vi "Load Sensors.vi"(8 "error in (no error)":errorcluster, 10 "refnum":T1, 11 "Sensor List Class in":refnum<class "Sensor List Class.lvclass">) -> (0 "error out":errorcluster, 2 "refnum out":T1, 3 "Sensor List Class out":refnum<class "Sensor List Class.lvclass">)   [LabVIEW 2013, in "Sensor List Class.lvclass"]
uses:
  Sensor List Class.lvclass
  <vilib>/Utility/config.llb/Config Data RefNum.ctl
  Sensor DAO Class.lvclass
  Sensor List Class.lvclass/Sensor List Class.ctl
  Sensor DAO Class.lvclass/Sensor DAO Class.ctl
  <vilib>/Utility/config.llb/NI_LVConfig.lvlib
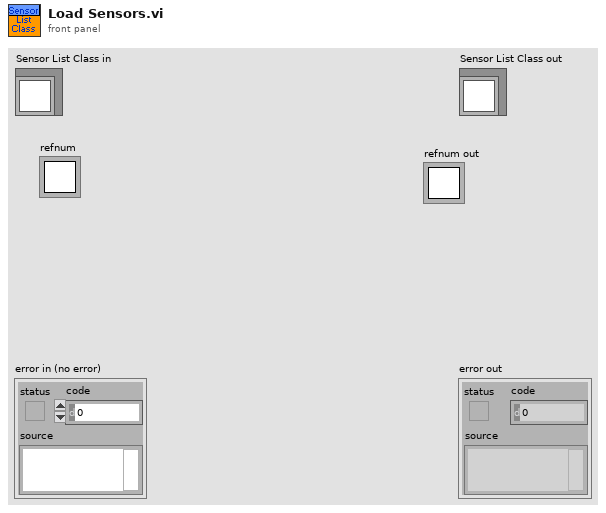
[diagram p1: front panel]
types:
  T1 = typedef "NI_LVConfig.lvlib/Config Data RefNum.ctl" = refnum<k1>
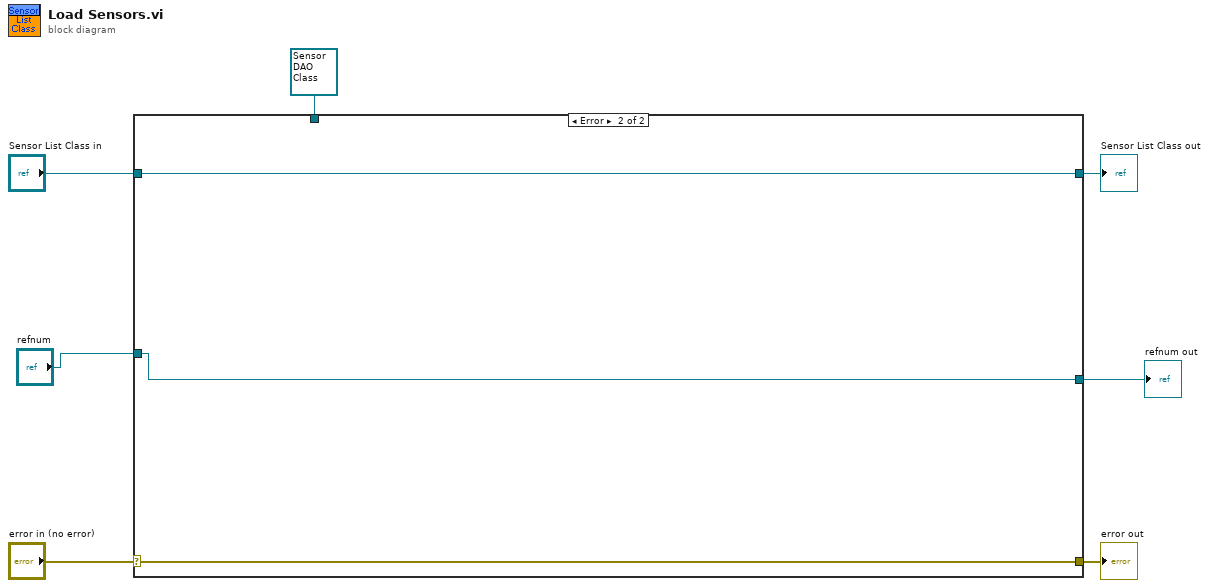
[diagram p0: block diagram]
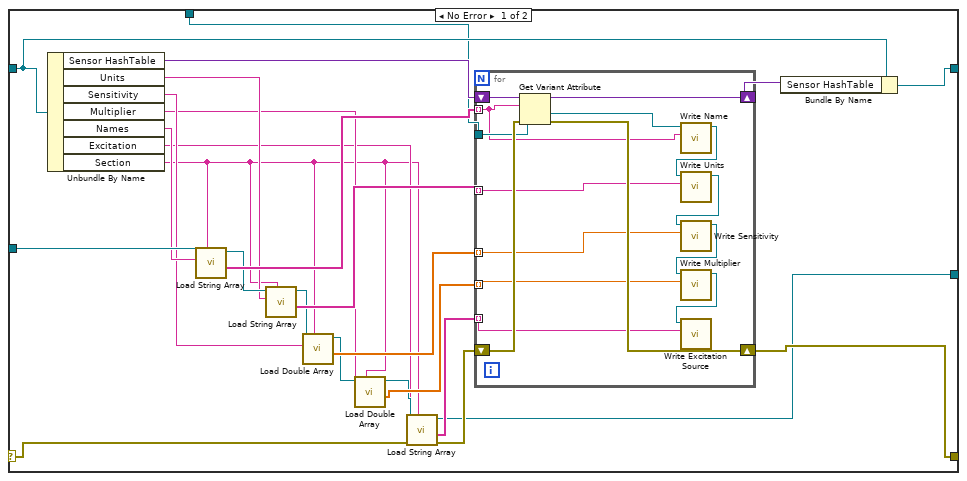
[diagram p2: hidden frame]
diagram:
  n1 = case shown="Error" "error in (no error)" {
    selector: "error in (no error)" -> [w22 w50]
    tunnel: [w21 w50] -> w6
    tunnel: [w18 w49] -> w4
    tunnel: "Sensor List Class in" -> [w20 w49]
    tunnel: "refnum" -> [w15 w48]
    tunnel: [w14 w48] -> w2
    tunnel: refnum<class "Sensor DAO Class.lvclass"> refnum ("Sensor DAO In") -> [w9 _]
    frame No Error {
      n2 = Unbundle By Name(w20) -> ("Sensor HashTable"=w19:variant, "Units"=w16:string, "Sensitivity"=w12:string, "Multiplier"=w11:string, "Names"=w13:string, "Excitation"=w10:string, "Section"=w8:string)
      n3 = call "Load String Array.vi"("section"=w8, "key"=w13, "refnum"=w15) -> ("String Array Out"=w27:string[], "refnum out"=w23:T1)  [unwired: 6 in, 1 out]
      n4 = call "Load String Array.vi"("section"=w8, "key"=w16, "refnum"=w23) -> ("String Array Out"=w28:string[], "refnum out"=w24:T1)  [unwired: 6 in, 1 out]
      n5 = call "Load Double Array.vi"("section"=w8, "key"=w12, "refnum"=w24) -> ("String Array Out"=w29:dbl[], "refnum out"=w25:T1)  [unwired: 6 in, 1 out]
      n6 = call "Load Double Array.vi"("section"=w8, "key"=w11, "refnum"=w25) -> ("String Array Out"=w30:dbl[], "refnum out"=w26:T1)  [unwired: 6 in, 1 out]
      n7 = call "Load String Array.vi"("section"=w8, "error in (no error)"=w22, "key"=w10, "refnum"=w26) -> ("error out"=w32:errorcluster, "String Array Out"=w31:string[], "refnum out"=w14:T1)  [unwired: 5 in]
      n8 = for {
        shift-right: [w46] -> w17
        shift-left: w19 -> [w47]
        shift-right: [w43] -> w21
        shift-left: w32 -> [w44]
        tunnel: w27 -> [w40] mode=indexing
        tunnel: w9 -> [w42]
        tunnel: w28 -> [w41] mode=indexing
        tunnel: w29 -> [w39] mode=indexing
        tunnel: w30 -> [w38] mode=indexing
        tunnel: w31 -> [w37] mode=indexing
        n9 = Get Variant Attribute(Variant=w47, name=w40, default value (empty Variant)=w42, error in=w44) -> (duplicate Variant=w46:variant, value=w45:refnum<class "Sensor DAO Class.lvclass">, error out=w43:errorcluster)  [unwired: 1 out]
        n10 = call "Write Name.vi"("Name"=w40, "Sensor DAO Class in"=w45) -> ("Sensor DAO Class out"=w36:refnum<class "Sensor DAO Class.lvclass">)  [unwired: 8 in, 1 out]
        n11 = call "Write Units.vi"("Units"=w41, "Sensor DAO Class in"=w36) -> ("Sensor DAO Class out"=w35:refnum<class "Sensor DAO Class.lvclass">)  [unwired: 8 in, 1 out]
        n12 = call "Write Sensitivity.vi"("Sensitivity"=w39, "Sensor DAO Class in"=w35) -> ("Sensor DAO Class out"=w34:refnum<class "Sensor DAO Class.lvclass">)  [unwired: 8 in, 1 out]
        n13 = call "Write Multiplier.vi"("Multiplier"=w38, "Sensor DAO Class in"=w34) -> ("Sensor DAO Class out"=w33:refnum<class "Sensor DAO Class.lvclass">)  [unwired: 8 in, 1 out]
        n14 = call "Write Excitation Source.vi"("Excitation Source"=w37, "Sensor DAO Class in"=w33) -> ()  [unwired: 8 in, 2 out]
      }
      n15 = Bundle By Name(cluster=w20, "Sensor HashTable"=w17) -> (w18:refnum<class "Sensor List Class.lvclass">)
    }
    frame Error {
    }
  }
  "error out" <- w6
  "Sensor List Class out" <- w4
  "refnum out" <- w2
